vi "labview_robotlimbleftjoint_command_mode_Server.vi"() -> ()   [LabVIEW 2010]
doc: "Template server that runs individual ros topics, services, etc. This is cloned for each topic being run."
uses:
  <userlib>/ROSforLV_0.1/ROS/Code/SubVIs/_ROSControl.ctl
  <userlib>/ROSforLV_0.1/ROS/Code/SubVIs/_ROSDirection.ctl
  <userlib>/ROSforLV_0.1/ROS/Code/_ROSDefinition.vi
panel:
  out "str to write":string
  out "Connected?":bool
  out "Specs":T2={"Server"="", "Node"="/labview", "Server Port"=5000, "URI (Subsc)"="", "Direction"=enum."Node"}
  out "Service Reply":string
  out "unregister":string="<?xml version='1.0'?>\n<methodResponse>\n<params>\n<param>\n<value><array><data>\n<value><int>1</int></value>\n<value><string>Registered [/labview] as publisher of [/robot/head/command_head_nod]</string></value>\n<value><array><data>\n<value><string>http://tuftsBaxter.local:56995/</string></value>\n</data></array></value>\n</data></array></value>\n</param>\n</params>\n</methodResponse>\n"
  out "Registered?":bool
  out "Requests":T3(array[cluster])
  out "Last Reply":string
  in  "stop":bool
  out "error out":errorcluster
  out "Connections":T4(array[cluster])
  in  "Baxter":T5
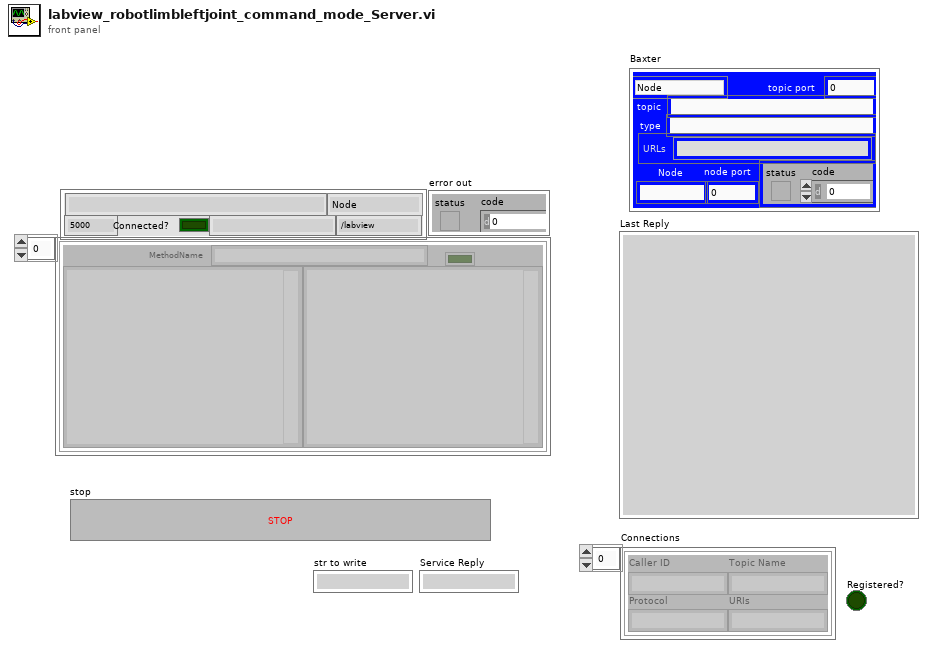
[diagram p1: front panel]
types:
  T1 = typedef "_ROSDirection.ctl" = enum16{"Node", "Publisher", "Subscriber", "Service Client"}
  T2 = cluster{"Server":string, "Node":string, "Server Port":u32, "URI (Subsc)":string, "Direction":T1}
  T3 = cluster{"First":string, "Second":string, "MethodName":string, "success":bool, "Dir1":string, "Dir2":string}[]
  T4 = cluster{"Caller ID":string, "Topic Name":string, "Protocol":string, "URIs":string}[]
  T5 = typedef "_ROSControl.ctl" = cluster{"topic port":u16, "Node":string, "topic":string, "type":string, "node port":u32, "error ":errorcluster, "Direction":T1, "APIs":string[]}
  T6 = cluster{"data out":string, "data out 2":string, "data out 3":string, "Success?":bool, "data out 4":string, "data out 5":string}[]
  T7 = cluster{"Code":i32, "Status Message":string, "APIs":string[]}
  T8 = cluster{"Server":string, "Node":string, "Server Port":u32, "URI (Subsc)":string, "connection":refnum<k5>, "Direction":T1}
  T9 = cluster{"Caller ID":string, "Topic Name":string, "Protocol":string, "URIs":string}
  T10 = cluster{"Protocol":string, "Code":i32, "IP":string, "Port":i32}
  T11 = cluster{"Node":string, "topic":string, "topic":string, "topic":string}
  T12 = cluster{"Code":i8, "statusMessage":string, "APIs":string[]}
  T13 = cluster{string, "data out":string, "Node":string, bool, string, string}
  T14 = cluster{"str to write":string, string, string, bool, string, string}
  T15 = cluster{string, string, string, bool, string, string}
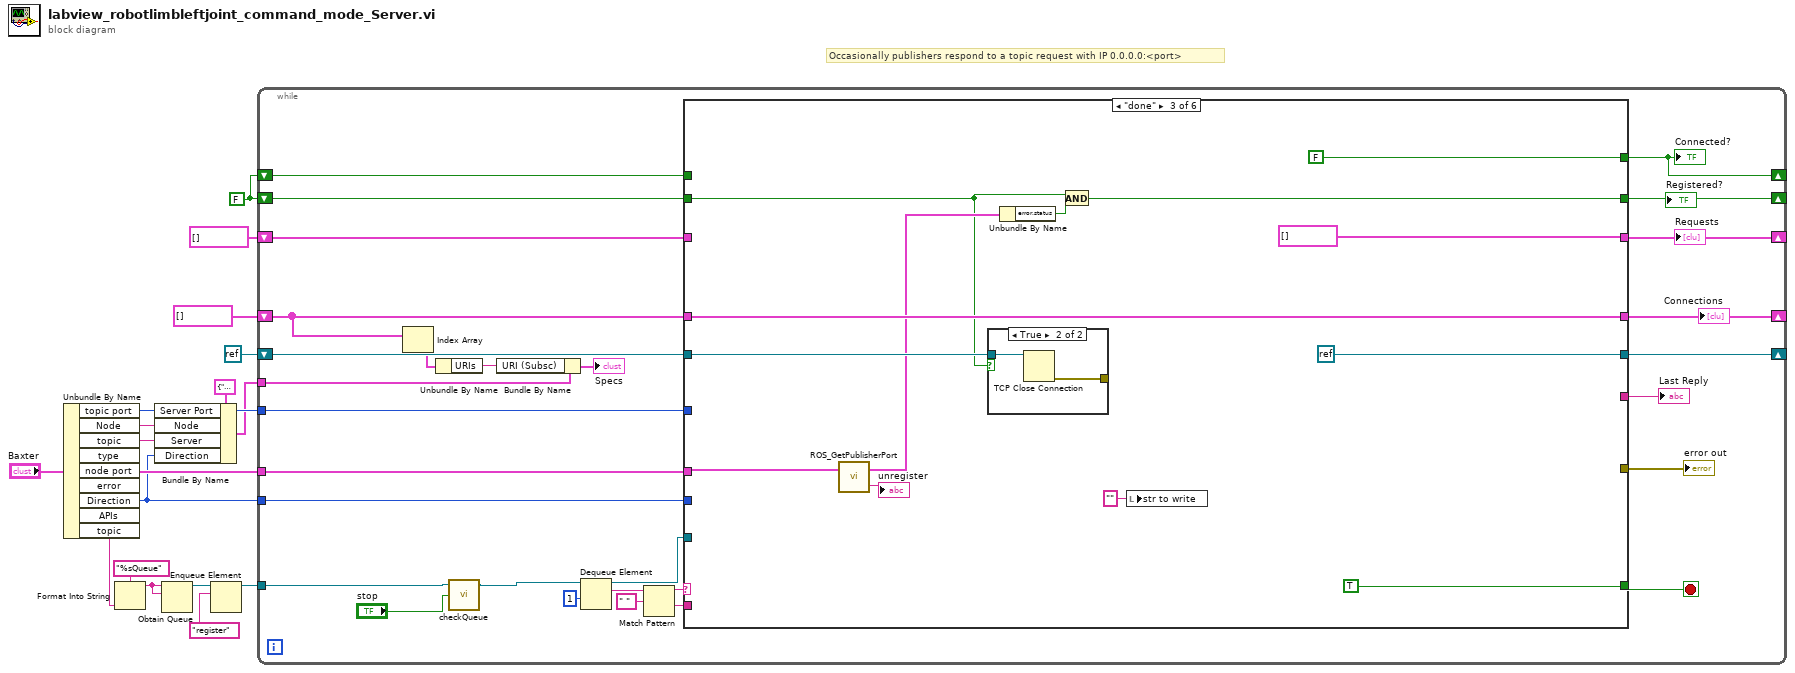
[diagram p0: block diagram]
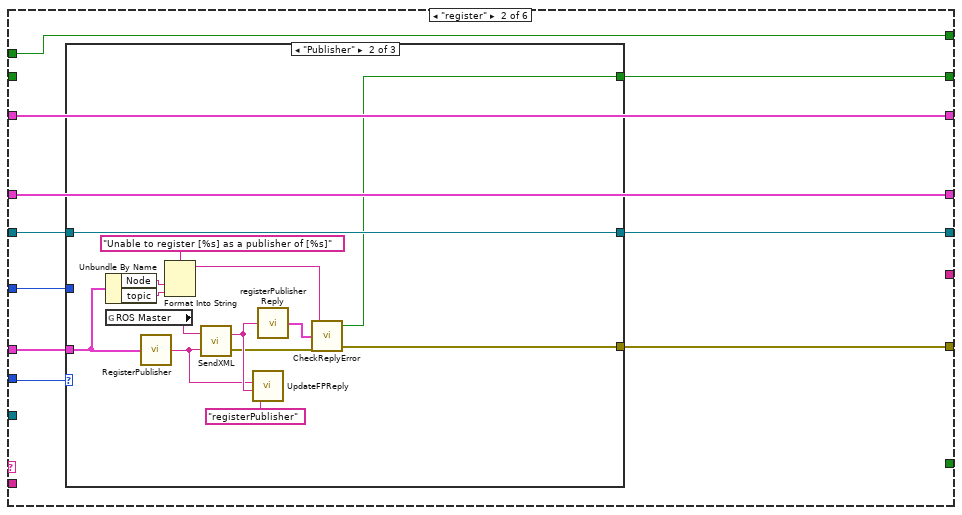
[diagram p3: hidden frame]
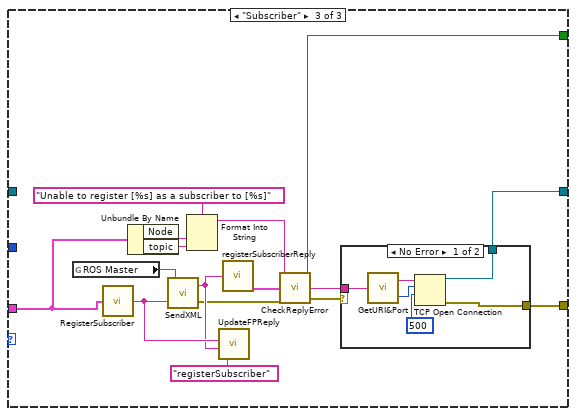
[diagram p5: hidden frame]
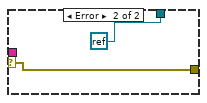
[diagram p6: hidden frame]
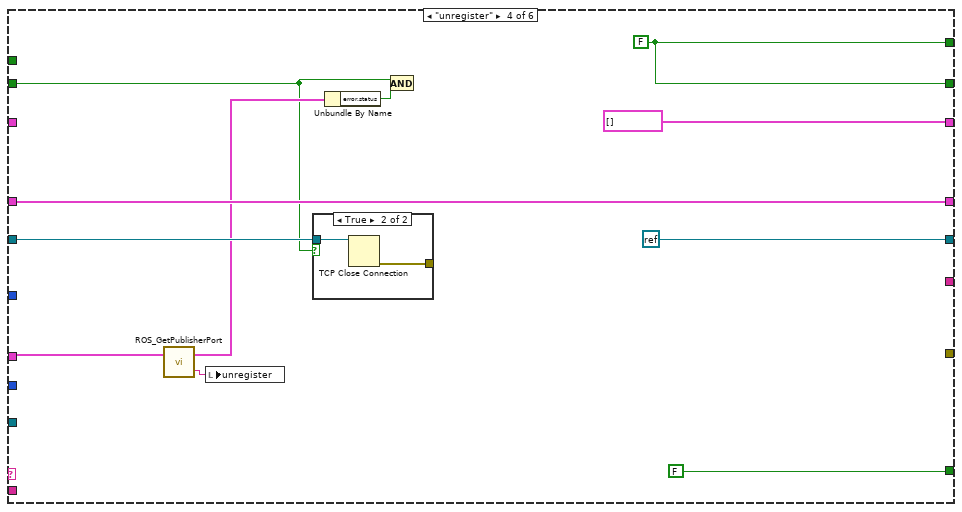
[diagram p8: hidden frame]
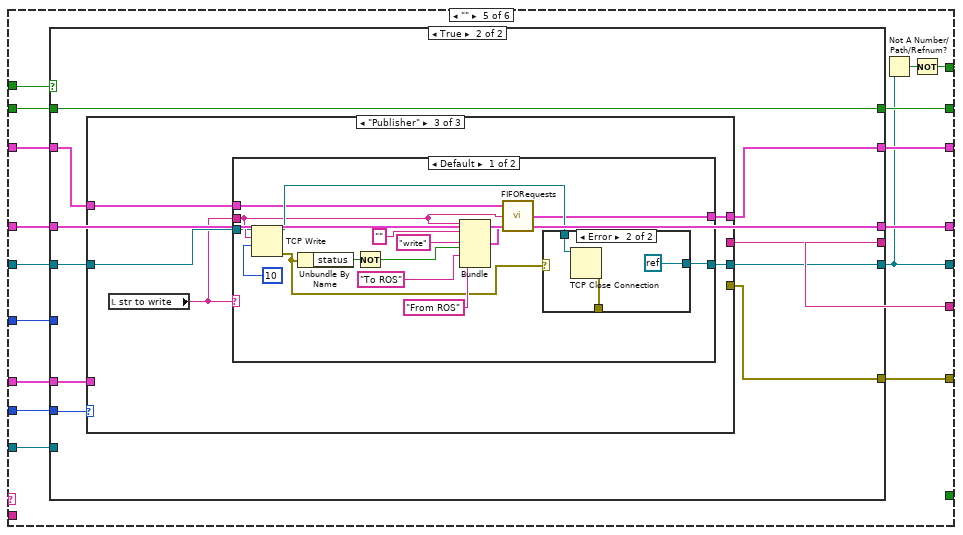
[diagram p10: hidden frame]
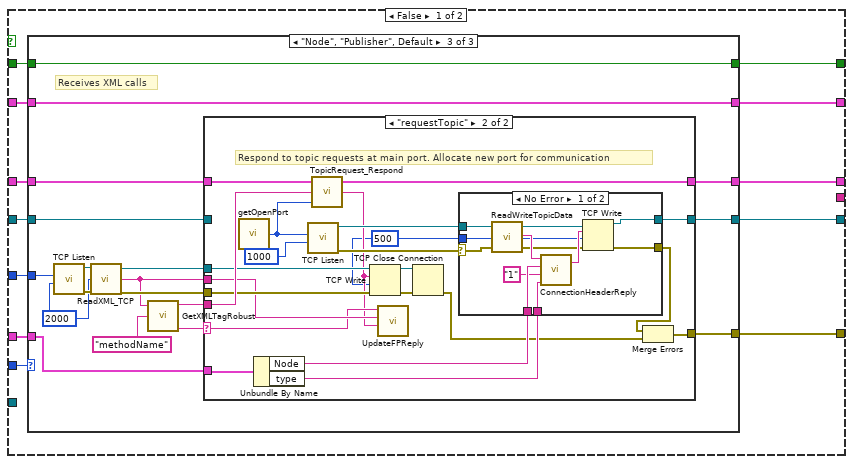
[diagram p11: hidden frame]
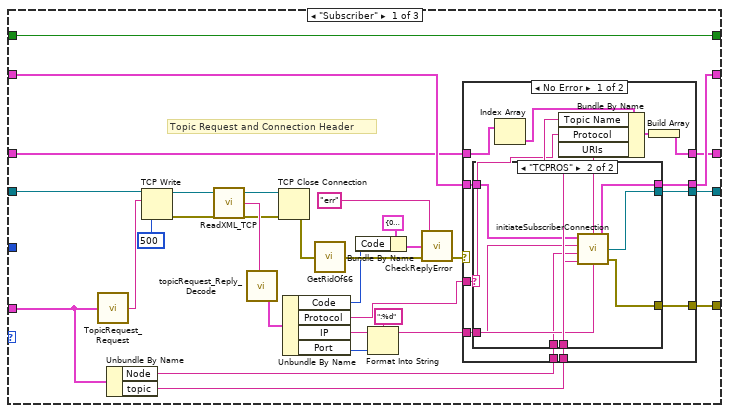
[diagram p12: hidden frame]
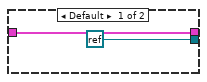
[diagram p13: hidden frame]
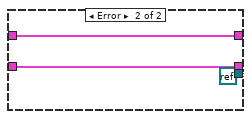
[diagram p14: hidden frame]
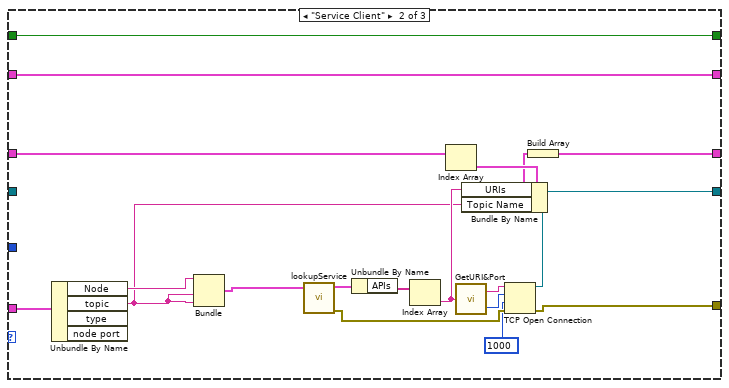
[diagram p15: hidden frame]
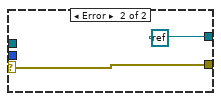
[diagram p17: hidden frame]
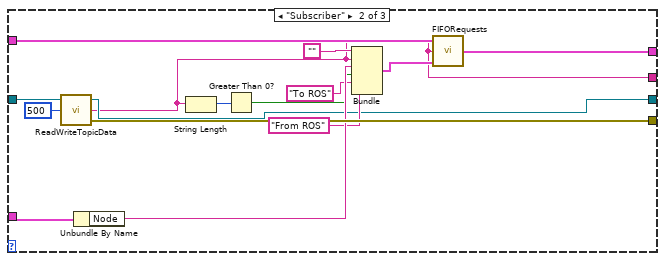
[diagram p19: hidden frame]
diagram:
  w12 = FALSE
  # "Occasionally publishers respond to a topic request with IP 0.0.0.0:<port>"
  n1 = Unbundle By Name("Baxter") -> ("topic port"=w6:u16, "Node"=w5:string, "topic"=w4:string, "Direction"=w3:T1, "topic"=w1:string)  [unwired: 4 out]
  n2 = Format Into String(format string="%sQueue", w1) -> (resulting string=w16:string)  [unwired: 2 in, 1 out]
  n3 = Bundle By Name(cluster=T2 {"Server"="", "Node"="/labview", "Server Port"=5000, "URI (Subsc)"="", "Direction"=enum."Node"} ("Specs"), "Server Port"=w6, "Node"=w5, "Server"=w4, "Direction"=w3) -> (w2:T2)
  n4 = Obtain Queue(name (unnamed)=w16, element data type=w16) -> (queue out=w9:refnum<queue>)  [unwired: 3 in, 2 out]
  n5 = Enqueue Element(queue=w9, element="register") -> (queue out=w8:refnum<queue>)  [unwired: 2 in, 2 out]
  n6 = while {
    tunnel: w6 -> [w46]
    shift-right: [w28] -> _
    shift-left: T4 [] ("Connections") -> [w26]
    shift-right: [w42] -> _
    shift-left: w12 -> [w45]
    shift-right: [w33] -> _
    shift-left: refnum<k0> refnum -> [w43]
    tunnel: w3 -> [w44]
    tunnel: "Baxter" -> [w41]
    tunnel: w8 -> [w20]
    shift-right: [w34] -> _
    shift-left: T6 [] ("Requests In") -> [w35]
    shift-right: [w30] -> _
    shift-left: w12 -> [w31]
    tunnel: w2 -> [w24]
    stop <- w32 stop-if-true
    n7 = Index Array(array=w26) -> (element=w25:T9)  [unwired: 1 in]
    n8 = Unbundle By Name(w25) -> ("URIs"=w23:string)
    n9 = call <userlib>:"checkQueue.vi"("stop"="stop", "queue in"=w20) -> ("queue out"=w19:refnum<queue>)  [unwired: 3 in]
    n10 = Bundle By Name(cluster=w24, "URI (Subsc)"=w23) -> (→"Specs":T2)
    n11 = Dequeue Element(queue=w19, timeout in ms (-1)=1) -> (queue out=w21:refnum<queue>, element=w39:string)  [unwired: 1 in, 2 out]
    n12 = Match Pattern(string=w39, regular expression=" ") -> (before substring=w37:string, after substring=w36:string)  [unwired: 1 in, 2 out]
    n13 = case shown="\"done\"" w37 {
      tunnel: w46 -> [_ w60 _ _ w145 _]
      tunnel: w26 -> [w51 w54 w111 w124 w144 w355]
      tunnel: [w51 w54 w111 w124 w143 w355] -> w28
      tunnel: w45 -> [w49 _ w103 w119 w135 w356]
      tunnel: w44 -> [_ w61 _ _ w142 w345]
      tunnel: [w50 w57 refnum<k0> refnum refnum<k0> refnum w133 w348] -> w33
      tunnel: w43 -> [w50 w56 w113 w126 w136 w354]
      tunnel: [w49 w53 w105 w117 w141 w356] -> w42
      tunnel: w41 -> [_ w59 w110 w123 w140 w343]
      tunnel: w36 -> [_ _ _ _ _ w352]
      tunnel: [_ _ TRUE FALSE _ _] -> w32
      tunnel: [_ w58 _ _ w137 w349] -> w29
      tunnel: w35 -> [w48 w55 _ _ w139 w351]
      tunnel: [w48 w55 T6 [] ("Requests Out") T6 [] ("Requests Out") w138 w350] -> w34
      tunnel: w31 -> [w47 w52 _ _ w134 w353]
      tunnel: [w47 w52 FALSE w117 w131 w346] -> w30
      tunnel: [_ _ _ _ w130 w344] -> w27
      tunnel: w21 -> [_ _ _ _ w129 w342]
      frame Default {
      }
      frame "register" {
        n14 = case shown="\"Publisher\"" w61 {
          tunnel: w60 -> [_ _ _]
          tunnel: w59 -> [_ w70 w83]
          tunnel: [_ w63 w80] -> w58
          tunnel: [w62 w68 w81] -> w57
          tunnel: w56 -> [w62 w68 _]
          tunnel: [_ w64 w77] -> w53
          frame "Node", Default {
          }
          frame "Publisher" {
            n15 = Unbundle By Name(w70) -> ("Node"=w72:string, "topic"=w71:string)
            n16 = global read "_ROSDefinition.vi" "ROS Master"() -> (w76:string)
            n17 = call <userlib>:"RegisterPublisher.vi"("ROS"=w70) -> ("XML"=w69:string)
            n18 = Format Into String(format string="Unable to register [%s] as a publisher of [%s]", w72, w71) -> (resulting string=w66:string)  [unwired: 2 in, 1 out]
            n19 = call <userlib>:"SendXML.vi"("Send"=w69, "URI in"=w76) -> ("error out"=w65:errorcluster, "Reply"=w75:string)
            n20 = call <userlib>:"UpdateFPReply.vi"("Reply"=w75, "Sent"=w69, "method"="registerPublisher") -> ()  [unwired: 3 in]
            n21 = call <userlib>:"registerPublisherReply.vi"("Response"=w75) -> ("Response"=w67:T7)
            n22 = call <userlib>:"CheckReplyError.vi"("error in"=w65, "Response"=w67, "Error String"=w66) -> ("error out"=w63:errorcluster, "Registered?"=w64:bool)  [unwired: 1 out]
          }
          frame "Subscriber" {
            n23 = global read "_ROSDefinition.vi" "ROS Master"() -> (w92:string)
            n24 = call <userlib>:"RegisterSubscriber.vi"("ROS"=w83) -> ("XML"=w90:string)
            n25 = Unbundle By Name(w83) -> ("Node"=w87:string, "topic"=w86:string)
            n26 = call <userlib>:"SendXML.vi"("Send"=w90, "URI in"=w92) -> ("error out"=w79:errorcluster, "Reply"=w89:string)
            n27 = Format Into String(format string="Unable to register [%s] as a subscriber to [%s]", w87, w86) -> (resulting string=w84:string)  [unwired: 2 in, 1 out]
            n28 = call <userlib>:"UpdateFPReply.vi"("Reply"=w89, "Sent"=w90, "method"="registerSubscriber") -> ()  [unwired: 3 in]
            n29 = call <userlib>:"registerSubscriberReply.vi"("Response"=w89) -> ("Response"=w88:T7)
            n30 = call <userlib>:"CheckReplyError.vi"("error in"=w79, "Response"=w88, "Error String"=w84) -> ("error out"=w78:errorcluster, "URI"=w82:string, "Registered?"=w77:bool)
            n31 = case shown="No Error" w78 {
              selector: w78 -> [_ w100]
              tunnel: w82 -> [w98 _]
              tunnel: [w94 refnum<k0> refnum] -> w81
              tunnel: [w93 w100] -> w80
              frame No Error {
                n32 = call <userlib>:"GetURI&Port.vi"("URI in"=w98) -> ("Port"=w96:u16, "URI"=w97:string)
                n33 = TCP Open Connection(address=w97, remote port or service name=w96, timeout ms (60000)=500) -> (connection ID=w94:refnum<k5>, error out=w93:errorcluster)  [unwired: 2 in]
              }
              frame Error {
              }
            }
          }
        }
      }
      frame "done" {
        n34 = call <userlib>:"ROS_GetPublisherPort.vi"("ROS in"=w110) -> ("Response"=→"unregister":string, "ROS out"=w107:T5)  [unwired: 1 in]
        n35 = case shown="True" w103 {
          tunnel: w113 -> [_ w115]
          tunnel: [_ w114] -> _
          frame False {
          }
          frame True {
            n36 = TCP Close Connection(connection ID=w115) -> (error out=w114:errorcluster)  [unwired: 2 in, 1 out]
          }
        }
        n37 = Unbundle By Name(w107) -> ("error.status"=w104:bool)
        n38 = And(x=w103, y=w104) -> (x .and. y?=w105:bool)
        n39 = local write "str to write"("" ("str to write")) -> ()
      }
      frame "unregister" {
        w117 = FALSE
        n40 = call <userlib>:"ROS_GetPublisherPort.vi"("ROS in"=w123) -> ("Response"=w116:string, "ROS out"=w121:T5)  [unwired: 1 in]
        n41 = local write "unregister"(w116) -> ()
        n42 = case shown="True" w119 {
          tunnel: w126 -> [_ w128]
          tunnel: [_ w127] -> _
          frame False {
          }
          frame True {
            n43 = TCP Close Connection(connection ID=w128) -> (error out=w127:errorcluster)  [unwired: 2 in, 1 out]
          }
        }
        n44 = Unbundle By Name(w121) -> ("error.status"=w120:bool)
        n45 = And(x=w119, y=w120) -> ()  [unwired: 1 out]
      }
      frame "" {
        n46 = case shown="True" w134 {
          tunnel: w145 -> [w157 _]
          tunnel: w144 -> [w156 w297]
          tunnel: [w155 w297] -> w143
          tunnel: w142 -> [w154 w298]
          tunnel: [w153 w291] -> w133
          tunnel: w136 -> [w152 w296]
          tunnel: [w151 w290] -> w141
          tunnel: w140 -> [w150 w295]
          tunnel: w139 -> [w149 w294]
          tunnel: [w148 w293] -> w138
          tunnel: [w146 w292] -> w137
          tunnel: w135 -> [w147 w290]
          tunnel: [_ w289] -> w130
          tunnel: w129 -> [_ _]
          frame False {
            n47 = case shown="\"Node\", \"Publisher\", Default" w154 {
              tunnel: w157 -> [_ _ w235]
              tunnel: w156 -> [w166 w218 w246]
              tunnel: [w165 w216 w243] -> w155
              tunnel: [w170 w222 w242] -> w153
              tunnel: w152 -> [w188 _ w236]
              tunnel: [w171 w230 w238] -> w151
              tunnel: w147 -> [w171 w230 w238]
              tunnel: w150 -> [w176 w229 w241]
              tunnel: w149 -> [w174 w231 w239]
              tunnel: [w173 w231 w239] -> w148
              tunnel: [w172 w221 w237] -> w146
              frame "Subscriber" {
                # "Topic Request and Connection Header"
                n48 = call <userlib>:"TopicRequest_Request.vi"("ROS"=w176) -> ("XML"=w187:string)
                n49 = Unbundle By Name(w176) -> ("Node"=w175:string, "topic"=w169:string)
                n50 = TCP Write(connection ID=w188, data in=w187, 9:500 ("timeout ms (25000)")) -> (connection ID out=w186:refnum<k5>, error out=w185:errorcluster)  [unwired: 1 in, 1 out]
                n51 = call <userlib>:"ReadXML_TCP.vi"("error in"=w185, "connection ID in"=w186) -> ("error out"=w181:errorcluster, "data out"=w183:string, "connection ID out"=w182:refnum<k5>)  [unwired: 1 in]
                n52 = call <userlib>:"topicRequest_Reply_Decode.vi"("Topic Request Reply"=w183) -> ("Topic Request Reply"=w180:T10)
                n53 = TCP Close Connection(connection ID=w182, error in (no error)=w181) -> (error out=w179:errorcluster)  [unwired: 1 in, 1 out]
                n54 = Unbundle By Name(w180) -> ("Code"=w160:i32, "Protocol"=w168:string, "IP"=w164:string, "Port"=w177:i32)
                n55 = call <userlib>:"GetRidOf66.vi"("error in (no error)"=w179) -> ("error out"=w162:errorcluster)
                n56 = Bundle By Name(cluster=T7 {"Code"=0, "Status Message"="", "APIs"=[]} ("Response"), "Code"=w160) -> (w158:T7)
                n57 = Format Into String(format string=":%d", initial string=w164, w177) -> (resulting string=w167:string)  [unwired: 1 in, 1 out]
                n58 = call <userlib>:"CheckReplyError.vi"("error in"=w162, "Response"=w158, "Error String"="err" ("source")) -> ("error out"=w161:errorcluster)  [unwired: 2 out]
                n59 = case shown="No Error" w161 {
                  tunnel: w168 -> [w192 _]
                  tunnel: w167 -> [w191 _]
                  tunnel: w175 -> [w200 _]
                  tunnel: w169 -> [w193 _]
                  tunnel: w174 -> [w199 w210]
                  tunnel: [w198 w210] -> w173
                  tunnel: [w197 _] -> w172
                  tunnel: [w196 refnum<k0> refnum] -> w170
                  tunnel: w166 -> [w195 w211]
                  tunnel: [w189 w211] -> w165
                  frame No Error {
                    n60 = case shown="\"TCPROS\"" w192 {
                      tunnel: w191 -> [_ w209]
                      tunnel: w200 -> [_ w208]
                      tunnel: w193 -> [_ w207]
                      tunnel: w199 -> [w201 w203]
                      tunnel: [w201 w206] -> w198
                      tunnel: [_ w205] -> w197
                      tunnel: [refnum<k0> refnum w204] -> w196
                      frame Default {
                      }
                      frame "TCPROS" {
                        n61 = call <userlib>:"initiateSubscriberConnection.vi"("topic"=w207, "Node"=w208, "URI"=w209, "Requests In"=w203) -> ("error out"=w205:errorcluster, "connection ID out"=w204:refnum<k5>, "Requests Out"=w206:T6)
                      }
                    }
                    n62 = Index Array(array=w195) -> (element=w194:T9)  [unwired: 1 in]
                    n63 = Bundle By Name(cluster=w194, "Topic Name"=w193, "Protocol"=w192, "URIs"=w191) -> (w190:T9)
                    n64 = Build Array(w190) -> (w189:T4)
                  }
                  frame Error {
                  }
                }
              }
              frame "Service Client" {
                n65 = Unbundle By Name(w229) -> ("Node"=w228:string, "topic"=w214:string)  [unwired: 2 out]
                n66 = Bundle("Node"=w228, "topic"=w214, "topic"=w214, "topic"=w214) -> (w227:T11)  [unwired: 1 in]
                n67 = call <userlib>:"lookupService.vi"("Parameters"=w227) -> ("Reply"=w226:T12, "error out"=w215:errorcluster)  [unwired: 4 in, 2 out]
                n68 = Unbundle By Name(w226) -> ("APIs"=w225:string[])
                n69 = Index Array(array=w225) -> (element=w219:string)  [unwired: 1 in]
                n70 = Index Array(array=w218) -> (element=w220:T9)  [unwired: 1 in]
                n71 = call <userlib>:"GetURI&Port.vi"("URI in"=w219) -> ("Port"=w223:u16, "URI"=w224:string)
                n72 = Bundle By Name(cluster=w220, "URIs"=w219, "Topic Name"=w214) -> (w217:T9)
                n73 = TCP Open Connection(address=w224, remote port or service name=w223, timeout ms (60000)=1000, error in (no error)=w215) -> (connection ID=w222:refnum<k5>, error out=w221:errorcluster)  [unwired: 1 in]
                n74 = Build Array(w217) -> (w216:T4)
              }
              frame "Node", "Publisher", Default {
                w232 = 2000 ("timeout ms (wait forever: -1)")
                # "Receives XML calls"
                n75 = call <vilib>:"TCP Listen.vi"("timeout ms (wait forever: -1)"=w232, "port"=w235) -> ("error out"=w233:errorcluster, "connection ID"=w234:refnum<k5>)  [unwired: 6 in, 2 out]
                n76 = call <userlib>:"ReadXML_TCP.vi"("error in"=w233, "timeout ms (3000)"=w232, "connection ID in"=w234) -> ("error out"=w244:errorcluster, "data out"=w240:string, "connection ID out"=w245:refnum<k5>)
                n77 = call <userlib>:"GetXMLTagRobust.vi"("Tag"="methodName", "String"=w240) -> ("value"=w248:string, "String w/o Tag"=w247:string)  [unwired: 1 in, 2 out]
                n78 = case shown="\"requestTopic\"" w248 {
                  selector: w248 -> [_ w261]
                  tunnel: w247 -> [_ w274]
                  tunnel: w246 -> [w252 w258]
                  tunnel: w245 -> [_ w271]
                  tunnel: w244 -> [w250 w270]
                  tunnel: [w252 w272] -> w243
                  tunnel: [w251 w259] -> w242
                  tunnel: w236 -> [w251 _]
                  tunnel: w241 -> [_ w265]
                  tunnel: w240 -> [_ w262]
                  tunnel: [w250 w254] -> w237
                  frame "False", Default {
                  }
                  frame "requestTopic" {
                    w257 = 500 ("timeout ms (25000)")
                    # "Respond to topic requests at main port. Allocate new port for communication"
                    n79 = call <userlib>:"getOpenPort.vi"() -> ("port"=w273:u16)
                    n80 = Unbundle By Name(w265) -> ("Node"=w264:string, "type"=w263:string)
                    n81 = call <vilib>:"TCP Listen.vi"("timeout ms (wait forever: -1)"=1000, "port"=w273) -> ("error out"=w267:errorcluster, "connection ID"=w266:refnum<k5>)  [unwired: 6 in, 2 out]
                    n82 = call <userlib>:"TopicRequest_Respond.vi"("port"=w273, "XML"=w274, "Subscribers"=w258) -> ("Topic Request Reply"=w260:string, "Subscribers"=w272:T4)  [unwired: 1 in]
                    n83 = TCP Write(connection ID=w271, data in=w260, error in (no error)=w270, 9:w257) -> (connection ID out=w268:refnum<k5>, error out=w269:errorcluster)  [unwired: 1 out]
                    n84 = call <userlib>:"UpdateFPReply.vi"("Reply"=w260, "Sent"=w262, "method"=w261) -> ()  [unwired: 3 in]
                    n85 = TCP Close Connection(connection ID=w268, error in (no error)=w269) -> (error out=w256:errorcluster)  [unwired: 1 in, 1 out]
                    n86 = case shown="No Error" w267 {
                      selector: w267 -> [w285 w287]
                      tunnel: w266 -> [w286 _]
                      tunnel: w264 -> [w283 _]
                      tunnel: w263 -> [w281 _]
                      tunnel: [w278 refnum<k0> refnum] -> w259
                      tunnel: [w276 w287] -> w255
                      tunnel: w257 -> [w275 _]
                      frame No Error {
                        n87 = call <userlib>:"ReadWriteTopicData.vi"("error in (no error)"=w285, "timeout ms (1000)"=w275, "connection ID in"=w286) -> ("error out"=w277:errorcluster, "data out"=w284:string, "connection ID out"=w279:refnum<k5>)
                        n88 = call <userlib>:"ConnectionHeaderReply.vi"("type"=w281, "Latching"="1", "Caller ID"=w283, "TCPROS Connection Header"=w284) -> ("Connection Response"=w280:string)  [unwired: 1 in]
                        n89 = TCP Write(connection ID=w279, data in=w280, error in (no error)=w277, 9:w275) -> (connection ID out=w278:refnum<k5>, error out=w276:errorcluster)  [unwired: 1 out]
                      }
                      frame Error {
                      }
                    }
                    n90 = Merge Errors(w255, w256) -> (w254:errorcluster)
                  }
                }
              }
            }
          }
          frame True {
            n91 = case shown="\"Publisher\"" w298 {
              tunnel: w296 -> [w299 w315 w318]
              tunnel: w295 -> [_ w308 _]
              tunnel: w294 -> [w300 w313 w320]
              tunnel: [w300 w312 w319] -> w293
              tunnel: [_ w311 _] -> w292
              tunnel: [w299 w302 w317] -> w291
              tunnel: [_ w301 _] -> w289
              frame "Node", Default {
              }
              frame "Subscriber" {
                n92 = call <userlib>:"ReadWriteTopicData.vi"("timeout ms (1000)"=500, "connection ID in"=w315) -> ("error out"=w311:errorcluster, "data out"=w301:string, "connection ID out"=w302:refnum<k5>)  [unwired: 1 in]
                n93 = Unbundle By Name(w308) -> ("Node"=w307:string)
                n94 = String Length(string=w301) -> (length=w310:i32)
                n95 = Greater Than 0?(x=w310) -> (x > 0?=w306:bool)
                n96 = Bundle("", "data out"=w301, "Node"=w307, w306, "To ROS", "From ROS") -> (w303:T13)  [unwired: 1 in]
                n97 = call <userlib>:"FIFORequests.vi"("New One"=w303, "data out"=w301, "Requests In"=w313) -> ("Requests Out"=w312:T6)
              }
              frame "Publisher" {
                n98 = local read "str to write"() -> (w316:string)
                n99 = case shown="Default" w316 {
                  tunnel: w320 -> [w328 w341]
                  tunnel: [w327 w341] -> w319
                  tunnel: w318 -> [w324 w340]
                  tunnel: [w323 w340] -> w317
                  tunnel: w316 -> [w325 _]
                  frame Default {
                    n100 = TCP Write(connection ID=w324, data in=w325, 9:10 ("timeout ms (25000)")) -> (connection ID out=w329:refnum<k5>, error out=w322:errorcluster)  [unwired: 1 in, 1 out]
                    n101 = Unbundle By Name(w322) -> ("status"=w331:bool)
                    n102 = Not(x=w331) -> (.not. x?=w330:bool)
                    n103 = Bundle("str to write"=w325, "", "write", w330, "To ROS", "From ROS") -> (w332:T14)  [unwired: 1 in]
                    n104 = call <userlib>:"FIFORequests.vi"("New One"=w332, "data out"=w325, "Requests In"=w328) -> ("Requests Out"=w327:T6)
                    n105 = case shown="Error" w322 {
                      tunnel: w329 -> [w336 w339]
                      tunnel: [w336 refnum<k0> refnum] -> w323
                      tunnel: [_ w337] -> _
                      frame No Error {
                      }
                      frame Error {
                        n106 = TCP Close Connection(connection ID=w339) -> (error out=w337:errorcluster)  [unwired: 2 in, 1 out]
                      }
                    }
                  }
                  frame "" {
                  }
                }
              }
            }
          }
        }
        n107 = Not A Number/Path/Refnum?(number/path/refnum=w133) -> (NaN/Path/Refnum?=w132:bool)
        n108 = Not(x=w132) -> (.not. x?=w131:bool)
      }
      frame "write" {
        n109 = case shown="True" w353 {
          tunnel: w354 -> [w361 w371]
          tunnel: w352 -> [w358 w368]
          tunnel: w351 -> [w362 w370]
          tunnel: [w362 w369] -> w350
          tunnel: [w361 w366] -> w348
          tunnel: [_ w367] -> w349
          tunnel: w345 -> [_ w365]
          tunnel: [_ w364] -> w344
          tunnel: w343 -> [_ w363]
          tunnel: w342 -> [w360 _]
          frame False {
            n110 = Format Into String(format string="write %s", w358) -> (resulting string=w357:string)  [unwired: 2 in, 1 out]
            n111 = call <userlib>:"cleanQueue.vi"("String"=w357, "queue in"=w360) -> ()  [unwired: 1 in, 1 out]
          }
          frame True {
            n112 = case shown="\"Publisher\"" w365 {
              tunnel: w371 -> [w372 w393 w408]
              tunnel: w370 -> [w373 w391 w417]
              tunnel: [w373 w390 w416] -> w369
              tunnel: w368 -> [_ w378 w415]
              tunnel: [_ w382 w414] -> w367
              tunnel: [w372 w380 refnum<k0> refnum] -> w366
              tunnel: [_ _ w413] -> w364
              tunnel: w363 -> [_ _ w412]
              frame "Node", Default {
              }
              frame "Publisher" {
                n113 = Match Pattern(string=w378, regular expression=" ") -> (before substring=w374:string, after substring=w375:string)  [unwired: 1 in, 2 out]
                n114 = case shown="Default" w374 {
                  selector: w374 -> [w395 _ _]
                  tunnel: w375 -> [_ w397 w398]
                  tunnel: [w395 w397 w398] -> w377
                  tunnel: ["" "" w398] -> w376
                  frame Default {
                  }
                  frame "stop_cont" {
                  }
                  frame "cont" {
                  }
                }
                "str to write" <- w376
                n115 = TCP Write(connection ID=w393, data in=w377, 9:1000 ("timeout ms (25000)")) -> (connection ID out=w381:refnum<k5>, error out=w382:errorcluster)  [unwired: 1 in, 1 out]
                n116 = Unbundle By Name(w382) -> ("status"=w384:bool)
                n117 = Not(x=w384) -> (.not. x?=w383:bool)
                n118 = Bundle(w377, "", "write", w383, "To ROS", "From ROS") -> (w385:T15)  [unwired: 1 in]
                n119 = call <userlib>:"FIFORequests.vi"("New One"=w385, "data out"=w377, "Requests In"=w391) -> ("Requests Out"=w390:T6)
                n120 = case shown="Error" w382 {
                  tunnel: w381 -> [w399 w402]
                  tunnel: [w399 refnum<k0> refnum] -> w380
                  tunnel: [_ w400] -> _
                  frame No Error {
                  }
                  frame Error {
                    n121 = TCP Close Connection(connection ID=w402) -> (error out=w400:errorcluster)  [unwired: 2 in, 1 out]
                  }
                }
              }
              frame "Service Client" {
                n122 = Unbundle By Name(w412) -> ("topic"=w404:string, "Node"=w405:string, "APIs"=w410:string[], "Direction"=w403:T1)
                n123 = Index Array(array=w410) -> (element=w409:string)  [unwired: 1 in]
                n124 = Bundle By Name(cluster=T8 {"Server"="", "Node"="/labview", "Server Port"=5000, "URI (Subsc)"="", "connection"=refnum, "Direction"=enum."Node"} ("Specs"), "Server"=w404, "Node"=w405, "URI (Subsc)"=w409, "connection"=w408, "Direction"=w403) -> (w407:T8)
                n125 = call <userlib>:"ROS_Service_Setup.vi"("Specs"=w407, "Msg to Send"=w415, "Requests In"=w417) -> ("error out"=w414:errorcluster, "Reply"=w413:string, "Requests Out"=w416:T6)
                "Service Reply" <- w413
              }
            }
          }
        }
        n126 = Not A Number/Path/Refnum?(number/path/refnum=w348) -> (NaN/Path/Refnum?=w347:bool)
        n127 = Not(x=w347) -> (.not. x?=w346:bool)
      }
    }
    "error out" <- w29
    "Requests" <- w34
    "Registered?" <- w42
    "Connected?" <- w30
    "Connections" <- w28
    "Last Reply" <- w27
  }
